vi "emi_Variant Value from String.vi"(0 "Value":string, 7 "Anything":variant, 11 "error in(no error)":errorcluster) -> (8 "Anything & Value":variant, 15 "error out":errorcluster)   [LabVIEW 2011]
doc: "Take a variant of a simple data type, take a string with text representing a value of the same datatype, combine the two. Get a variant with the value the text represented.\n\nThis vi is designed spesificaly to interprat the text created by \"Simple Variant Info.vi\". It may be used with orther text data, but formating may be a problem.\n\nIntended use: Together with ini files and other text representations of values.\n\nSupports all data types except:\nVariant\nPicture\nTag\nArray\nWaveform\nDigital Waveform\nDigital Data\nExpressData\nRefnum\nExternal Data\nVI\nPoly VI\nLabview Class Instance\nFixed point\nCluster\n\nOn error: No operation"
uses:
  <vilib>/Utility/VariantDataType/UnitType.ctl
  <vilib>/Utility/VariantDataType/UnitInfo.ctl
  Error/emi_Create Error.vi
  <vilib>/Utility/VariantDataType/VariantType.lvlib
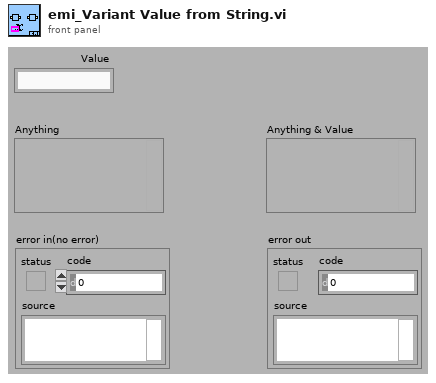
[diagram p1: front panel]
types:
  T1 = typedef "VariantType.lvlib/UnitInfo.ctl" = cluster{"UnitType":T2, "Exponent":i16}
  T2 = typedef "VariantType.lvlib/UnitType.ctl" = enum16{"Radians", "Steradians", "Seconds", "Meters", "Kilograms", "Amperes", "Kelvins", "Moles", "Candelas", "InvalidUnit"}
  T3 = typedef "VariantType.lvlib/Type.ctl" = enum8{"Invalid Type", "Void", "I8", "I16", "I32", "I64", "U8", "U16", "U32", "U64", "Single Float", "Double Float", "Extended Float", "Single Complex", "Double Complex", "Extended Complex", "Enum U8", "Enum U16", "Enum U32", "Enum U64", "Single Float With Unit", "Double Float With Unit", "Extended Float With Unit", "Single Complex with Unit", "Double Complex with Unit", "Extended Complex with Unit", "Boolean", "String", "Path", "Picture", "Tag", "Array", "Cluster", "Variant", "LV Variant", "Waveform", "Timestamp", "Digital Waveform", "Digital Data", "ExpressData", "Refnum", "External Data", "VI", "Poly VI", "LabVIEW Class Instance", "Fixed Point"}
  T4 = typedef "VariantType.lvlib/TypedefInfo.ctl" = cluster{"Name":string, "Timestamp":u32}
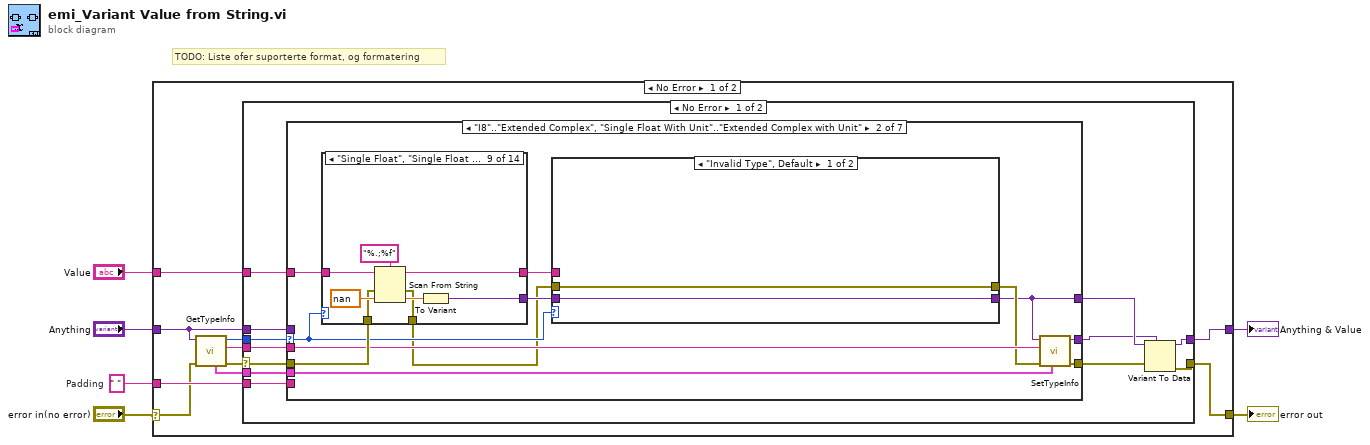
[diagram p0: block diagram]
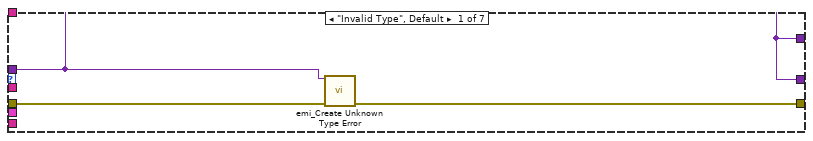
[diagram p2: hidden frame]
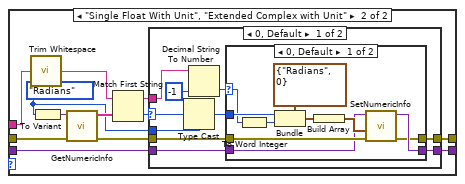
[diagram p3: hidden frame]
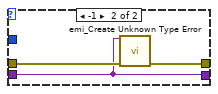
[diagram p4: hidden frame]
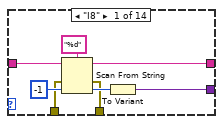
[diagram p6: hidden frame]
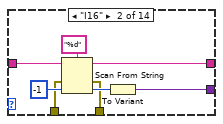
[diagram p7: hidden frame]
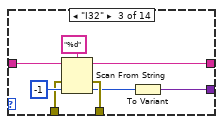
[diagram p8: hidden frame]
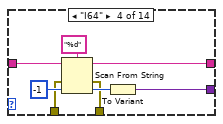
[diagram p9: hidden frame]
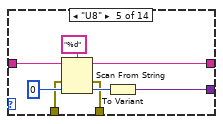
[diagram p10: hidden frame]
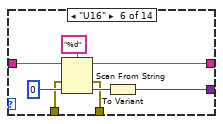
[diagram p11: hidden frame]
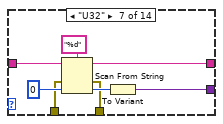
[diagram p12: hidden frame]
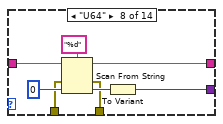
[diagram p13: hidden frame]
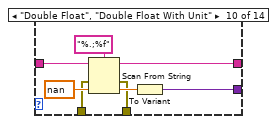
[diagram p14: hidden frame]
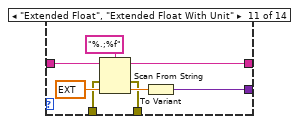
[diagram p15: hidden frame]
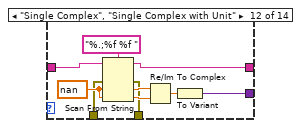
[diagram p16: hidden frame]
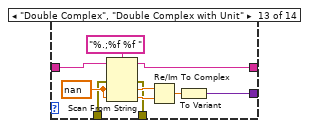
[diagram p17: hidden frame]
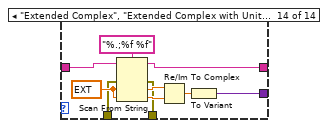
[diagram p18: hidden frame]
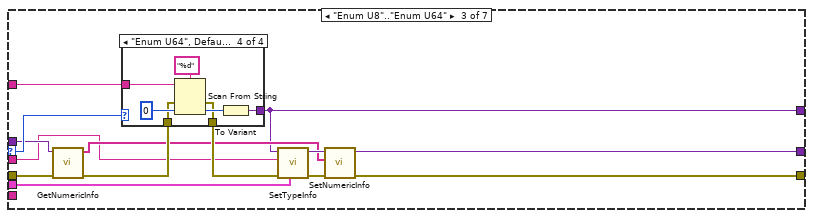
[diagram p19: hidden frame]
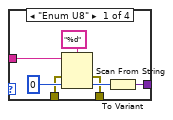
[diagram p20: hidden frame]
diagram:
  w4 = " "  # Padding
  # "TODO: Liste ofer suporterte format, og formatering"
  n1 = case shown="No Error" "error in(no error)" {
    selector: "error in(no error)" -> [w7 w283]
    tunnel: [w16 w283] -> w6
    tunnel: "Anything" -> [w14 w284]
    tunnel: w4 -> [w13 _]
    tunnel: "Value" -> [w12 _]
    tunnel: [w9 w284] -> w3
    frame No Error {
      n2 = call <vilib>:"GetTypeInfo.vi"("error in (no error)"=w7, "Variant"=w14) -> ("error out"=w8:errorcluster, "Name"=w11:string, "Type Enum"=w15:T3, "TypedefInfo"=w10:T4)  [unwired: 5 in, 1 out]
      n3 = case shown="No Error" w8 {
        selector: w8 -> [w23 w282]
        tunnel: [w21 w282] -> w16
        tunnel: w15 -> [w28 _]
        tunnel: w14 -> [w18 w281]
        tunnel: w13 -> [w27 _]
        tunnel: w12 -> [w26 _]
        tunnel: w11 -> [w25 _]
        tunnel: w10 -> [w24 _]
        tunnel: [w20 w281] -> w9
        frame No Error {
          n4 = case shown="\"I8\"..\"Extended Complex\", \"Single Float With Unit\"..\"Extended Complex with Unit\"" w28 {
            selector: w28 -> [_ w39 w212 _ _ _ _]
            tunnel: w18 -> [w29 _ w208 _ _ _ _]
            tunnel: w23 -> [w31 w42 w210 w248 w259 w270 w278]
            tunnel: [w30 w34 w204 w250 w265 w272 w280] -> w22
            tunnel: w27 -> [_ _ _ _ _ _ _]
            tunnel: w26 -> [_ w43 w213 w244 w262 w268 w276]
            tunnel: w25 -> [_ w41 w203 w249 w261 w271 w279]
            tunnel: w24 -> [_ w40 w211 w247 w260 w269 w277]
            tunnel: [w29 w33 w202 w246 w264 w267 w275] -> w17
            tunnel: [w29 w32 w201 w245 w263 w266 w273] -> w19
            frame "Invalid Type", Default {
              n5 = call "emi_Create Unknown Type Error.vi"("Anything"=w29, "error IO"=w31) -> ("error out"=w30:errorcluster)  [unwired: 13 in]
            }
            frame "I8".."Extended Complex", "Single Float With Unit".."Extended Complex with Unit" {
              n6 = case shown="\"Single Float\", \"Single Float With Unit\"" w39 {
                tunnel: w43 -> [w89 w97 w105 w113 w121 w129 w137 w145 w153 w161 w169 w173 w183 w193]
                tunnel: w42 -> [w87 w95 w103 w111 w119 w127 w135 w143 w151 w159 w167 w175 w185 w195]
                tunnel: [w85 w93 w102 w109 w117 w125 w133 w141 w149 w157 w165 w174 w184 w194] -> w37
                tunnel: [w84 w92 w101 w108 w116 w124 w132 w140 w148 w156 w164 w172 w182 w192] -> w38
                tunnel: [w83 w91 w100 w107 w115 w123 w131 w139 w147 w155 w163 w171 w181 w191] -> w35
                frame "I8" {
                  n7 = Scan From String(format string="%d", input string=w89, error in=w87, default 1=i8 -1) -> (remaining string=w83:string, error out=w85:errorcluster, output 1=w86:i8)  [unwired: 1 in, 1 out]
                  n8 = To Variant(anything=w86) -> (Variant=w84:variant)
                }
                frame "I16" {
                  n9 = Scan From String(format string="%d", input string=w97, error in=w95, default 1=i16 -1) -> (remaining string=w91:string, error out=w93:errorcluster, output 1=w94:i16)  [unwired: 1 in, 1 out]
                  n10 = To Variant(anything=w94) -> (Variant=w92:variant)
                }
                frame "I32" {
                  n11 = Scan From String(format string="%d", input string=w105, error in=w103, default 1=-1) -> (remaining string=w100:string, error out=w102:errorcluster, output 1=w99:i32)  [unwired: 1 in, 1 out]
                  n12 = To Variant(anything=w99) -> (Variant=w101:variant)
                }
                frame "I64" {
                  n13 = Scan From String(format string="%d", input string=w113, error in=w111, default 1=i64 -1) -> (remaining string=w107:string, error out=w109:errorcluster, output 1=w110:i64)  [unwired: 1 in, 1 out]
                  n14 = To Variant(anything=w110) -> (Variant=w108:variant)
                }
                frame "U8" {
                  n15 = Scan From String(format string="%d", input string=w121, error in=w119, default 1=u8 0) -> (remaining string=w115:string, error out=w117:errorcluster, output 1=w118:u8)  [unwired: 1 in, 1 out]
                  n16 = To Variant(anything=w118) -> (Variant=w116:variant)
                }
                frame "U16" {
                  n17 = Scan From String(format string="%d", input string=w129, error in=w127, default 1=u16 0) -> (remaining string=w123:string, error out=w125:errorcluster, output 1=w126:u16)  [unwired: 1 in, 1 out]
                  n18 = To Variant(anything=w126) -> (Variant=w124:variant)
                }
                frame "U32" {
                  n19 = Scan From String(format string="%d", input string=w137, error in=w135, default 1=u32 0) -> (remaining string=w131:string, error out=w133:errorcluster, output 1=w134:u32)  [unwired: 1 in, 1 out]
                  n20 = To Variant(anything=w134) -> (Variant=w132:variant)
                }
                frame "U64" {
                  n21 = Scan From String(format string="%d", input string=w145, error in=w143, default 1=u64 0) -> (remaining string=w139:string, error out=w141:errorcluster, output 1=w142:u64)  [unwired: 1 in, 1 out]
                  n22 = To Variant(anything=w142) -> (Variant=w140:variant)
                }
                frame "Single Float", "Single Float With Unit" {
                  n23 = Scan From String(format string="%.;%f", input string=w153, error in=w151, default 1=sgl nan) -> (remaining string=w147:string, error out=w149:errorcluster, output 1=w150:sgl)  [unwired: 1 in, 1 out]
                  n24 = To Variant(anything=w150) -> (Variant=w148:variant)
                }
                frame "Double Float", "Double Float With Unit" {
                  n25 = Scan From String(format string="%.;%f", input string=w161, error in=w159, default 1=nan) -> (remaining string=w155:string, error out=w157:errorcluster, output 1=w158:dbl)  [unwired: 1 in, 1 out]
                  n26 = To Variant(anything=w158) -> (Variant=w156:variant)
                }
                frame "Extended Float", "Extended Float With Unit" {
                  n27 = Scan From String(format string="%.;%f", input string=w169, error in=w167, default 1=ext nan) -> (remaining string=w163:string, error out=w165:errorcluster, output 1=w166:ext)  [unwired: 1 in, 1 out]
                  n28 = To Variant(anything=w166) -> (Variant=w164:variant)
                }
                frame "Single Complex", "Single Complex with Unit" {
                  w180 = sgl nan
                  n29 = Scan From String(format string="%.;%f %f ", input string=w173, error in=w175, default 1=w180, default 2=w180) -> (remaining string=w171:string, error out=w174:errorcluster, output 1=w177:sgl, output 2=w178:sgl)  [unwired: 1 in, 1 out]
                  n30 = Re/Im To Complex(1:w178, 2:w177) -> (0:w179:csg)
                  n31 = To Variant(anything=w179) -> (Variant=w172:variant)
                }
                frame "Double Complex", "Double Complex with Unit" {
                  w190 = nan
                  n32 = Scan From String(format string="%.;%f %f ", input string=w183, error in=w185, default 1=w190, default 2=w190) -> (remaining string=w181:string, error out=w184:errorcluster, output 1=w187:dbl, output 2=w188:dbl)  [unwired: 1 in, 1 out]
                  n33 = Re/Im To Complex(1:w188, 2:w187) -> (0:w189:cdb)
                  n34 = To Variant(anything=w189) -> (Variant=w182:variant)
                }
                frame "Extended Complex", "Extended Complex with Unit", Default {
                  w200 = ext nan
                  n35 = Scan From String(format string="%.;%f %f", input string=w193, error in=w195, default 1=w200, default 2=w200) -> (remaining string=w191:string, error out=w194:errorcluster, output 1=w197:ext, output 2=w198:ext)  [unwired: 1 in, 1 out]
                  n36 = Re/Im To Complex(1:w198, 2:w197) -> (0:w199:cxt)
                  n37 = To Variant(anything=w199) -> (Variant=w192:variant)
                }
              }
              n38 = case shown="\"Invalid Type\", Default" w39 {
                tunnel: w35 -> [_ w55]
                tunnel: w38 -> [w45 w48]
                tunnel: [w45 w49] -> w32
                tunnel: [w44 w47] -> w36
                tunnel: w37 -> [w44 w46]
                frame "Invalid Type", Default {
                }
                frame "Single Float With Unit", "Extended Complex with Unit" {
                  w51 = UnitType."Radians" ("UnitType")
                  n39 = call <vilib>:"Trim Whitespace.vi"("string"=w55) -> ("trimmed string"=w54:string)  [unwired: 1 in]
                  n40 = To Variant(anything=w51) -> (Variant=w56:variant)
                  n41 = call <vilib>:"GetNumericInfo.vi"("error in (no error)"=w46, "Variant"=w56) -> ("error out"=w50:errorcluster, "EnumNames"=w57:string[])  [unwired: 6 in, 2 out]
                  n42 = Match First String(2:w57, 3:w54) -> (0:w53:i32, 1:w52:string)
                  n43 = case shown="0, Default" w53 {
                    selector: w53 -> [w66 _]
                    tunnel: w52 -> [w65 _]
                    tunnel: w51 -> [w67 _]
                    tunnel: w50 -> [w63 w81]
                    tunnel: [w61 w82] -> w49
                    tunnel: w48 -> [w62 w82]
                    tunnel: [w60 w81] -> w47
                    frame 0, Default {
                      n44 = Type Cast(type=w67, x=w66) -> (*(type *) &x=w64:T2)
                      n45 = Decimal String To Number(string=w65, default (0L)=-1 ("default (0 I32)")) -> (number=w58:i32)  [unwired: 1 in, 1 out]
                      n46 = case shown="0, Default" w58 {
                        selector: w58 -> [w69 _]
                        tunnel: w64 -> [w76 _]
                        tunnel: w63 -> [w73 w80]
                        tunnel: w62 -> [w72 w78]
                        tunnel: [w71 w78] -> w61
                        tunnel: [w70 w79] -> w60
                        frame 0, Default {
                          n47 = To Word Integer(number=w69) -> (16bit integer=w68:i16)
                          n48 = Bundle(cluster=T1 {"UnitType"=enum."Radians", "Exponent"=0} ("Unit"), "UnitType"=w76, "Exponent"=w68) -> (w75:T1)
                          n49 = Build Array(w75) -> (w74:T1[])
                          n50 = call <vilib>:"SetNumericInfo.vi"("error in (no error)"=w73, "Units"=w74, "Variant"=w72) -> ("error out"=w70:errorcluster, "Variant Out"=w71:variant)  [unwired: 7 in]
                        }
                        frame -1 {
                          n51 = call "emi_Create Unknown Type Error.vi"("Anything"=w78, "error IO"=w80) -> ("error out"=w79:errorcluster)  [unwired: 13 in]
                        }
                      }
                    }
                    frame -1 {
                    }
                  }
                }
              }
              n52 = call <vilib>:"SetTypeInfo.vi"("Typedef Info"=w40, "error in (no error)"=w36, "Name"=w41, "Variant"=w32) -> ("error out"=w34:errorcluster, "Variant Out"=w33:variant)  [unwired: 6 in]
            }
            frame "Enum U8".."Enum U64" {
              n53 = call <vilib>:"GetNumericInfo.vi"("error in (no error)"=w210, "Variant"=w208) -> ("error out"=w209:errorcluster, "EnumNames"=w205:string[])  [unwired: 6 in, 2 out]
              n54 = case shown="\"Enum U64\", Default" w212 {
                tunnel: w213 -> [w220 w227 w234 w241]
                tunnel: w209 -> [w218 w225 w232 w239]
                tunnel: [w216 w223 w230 w237] -> w214
                tunnel: [w215 w222 w229 w236] -> w201
                frame "Enum U8" {
                  n55 = Scan From String(format string="%d", input string=w220, error in=w218, default 1=u8 0) -> (error out=w216:errorcluster, output 1=w217:u8)  [unwired: 1 in, 2 out]
                  n56 = To Variant(anything=w217) -> (Variant=w215:variant)
                }
                frame "Enum U16" {
                  n57 = Scan From String(format string="%d", input string=w227, error in=w225, default 1=u16 0) -> (error out=w223:errorcluster, output 1=w224:u16)  [unwired: 1 in, 2 out]
                  n58 = To Variant(anything=w224) -> (Variant=w222:variant)
                }
                frame "Enum U32" {
                  n59 = Scan From String(format string="%d", input string=w234, error in=w232, default 1=u32 0) -> (error out=w230:errorcluster, output 1=w231:u32)  [unwired: 1 in, 2 out]
                  n60 = To Variant(anything=w231) -> (Variant=w229:variant)
                }
                frame "Enum U64", Default {
                  n61 = Scan From String(format string="%d", input string=w241, error in=w239, default 1=u64 0) -> (error out=w237:errorcluster, output 1=w238:u64)  [unwired: 1 in, 2 out]
                  n62 = To Variant(anything=w238) -> (Variant=w236:variant)
                }
              }
              n63 = call <vilib>:"SetTypeInfo.vi"("Typedef Info"=w211, "error in (no error)"=w214, "Name"=w203, "Variant"=w201) -> ("error out"=w207:errorcluster, "Variant Out"=w206:variant)  [unwired: 6 in]
              n64 = call <vilib>:"SetNumericInfo.vi"("error in (no error)"=w207, "Enum Names"=w205, "Variant"=w206) -> ("error out"=w204:errorcluster, "Variant Out"=w202:variant)  [unwired: 7 in]
            }
            frame "Boolean" {
              n65 = To Lower Case(string=w244) -> (all lower case string=w243:string)
              n66 = call <vilib>:"Trim Whitespace.vi"("string"=w243) -> ("trimmed string"=w254:string)  [unwired: 1 in]
              n67 = Match True/False String(2:"false", 3:"true", 4:w254) -> (0:w251:bool)  [unwired: 1 out]
              n68 = To Variant(anything=w251) -> (Variant=w245:variant)
              n69 = call <vilib>:"SetTypeInfo.vi"("Typedef Info"=w247, "error in (no error)"=w248, "Name"=w249, "Variant"=w245) -> ("error out"=w250:errorcluster, "Variant Out"=w246:variant)  [unwired: 6 in]
            }
            frame "Timestamp" {
              n70 = call <vilib>:"Trim Whitespace.vi"("string"=w262) -> ("trimmed string"=w257:string)  [unwired: 1 in]
              n71 = Scan From String(format string="%^<%Y%m%d %H%M%S%6u>T", input string=w257, error in=w259) -> (error out=w258:errorcluster, output 1=w255:timestamp)  [unwired: 2 in, 2 out]
              n72 = To Variant(anything=w255) -> (Variant=w263:variant)
              n73 = call <vilib>:"SetTypeInfo.vi"("Typedef Info"=w260, "error in (no error)"=w258, "Name"=w261, "Variant"=w263) -> ("error out"=w265:errorcluster, "Variant Out"=w264:variant)  [unwired: 6 in]
            }
            frame "String" {
              n74 = To Variant(anything=w268) -> (Variant=w266:variant)
              n75 = call <vilib>:"SetTypeInfo.vi"("Typedef Info"=w269, "error in (no error)"=w270, "Name"=w271, "Variant"=w266) -> ("error out"=w272:errorcluster, "Variant Out"=w267:variant)  [unwired: 6 in]
            }
            frame "Path" {
              n76 = String To Path(string=w276) -> (path=w274:path)
              n77 = To Variant(anything=w274) -> (Variant=w273:variant)
              n78 = call <vilib>:"SetTypeInfo.vi"("Typedef Info"=w277, "error in (no error)"=w278, "Name"=w279, "Variant"=w273) -> ("error out"=w280:errorcluster, "Variant Out"=w275:variant)  [unwired: 6 in]
            }
          }
          n79 = Variant To Data(error in=w22, type=w17, Variant=w19) -> (data=w20:variant, error out=w21:errorcluster)
        }
        frame Error {
        }
      }
    }
    frame Error {
    }
  }
  "error out" <- w6
  "Anything & Value" <- w3
